vi "FIU Global Strings.vi"() -> ()   [LabVIEW 2011, in "PXI-2514 Custom Device.lvlib"]
uses:
  PXI-2514 Custom Device.lvlib
panel:
  in  "Fault Channel Description":string="The \"Name (Alias)\" for each channel may be changed. The \"Hardware Channel #\" cannot be changed by the user, and represents the actual Fault Channel being controller.\n\nThe Fault Default Value sets the default state for the channel."
  in  "Channel Fault":string="Channel Fault"
  in  "FIU Channel #":string="FIU Channel #"
  in  "Hardware Device Name":string="Hardware Device Name"
  in  "FIU Description":string="This is a Custom Device for the PXI-2514 FIU."
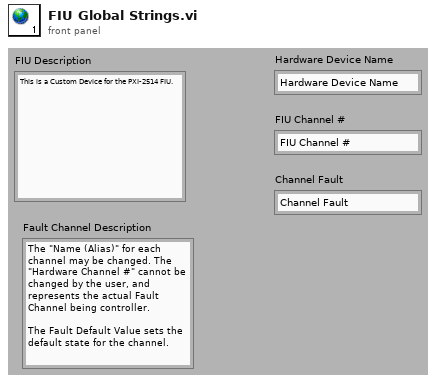
[diagram p1: front panel]
diagram:
